vi "Config Display Font Size.vi"() -> ()   [LabVIEW 2016]
panel:
  in  "Font Size And Precision":T1={"Channel Font Size"=0, "Channel Value Font Size"=0, "Unit Font Size"=0, "Row Font Size"=0, "Display Precision"=2}
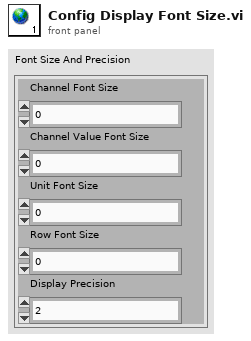
[diagram p1: front panel]
types:
  T1 = cluster{"Channel Font Size":u32, "Channel Value Font Size":u32, "Unit Font Size":u32, "Row Font Size":u32, "Display Precision":u32}
diagram:
